vi "XML_value_to_variant.vi"(0 "XML-param":string) -> (1 "ParsingErrors":string, 2 "Value":variant, 3 "Type":T1(ring))   [LabVIEW 2010]
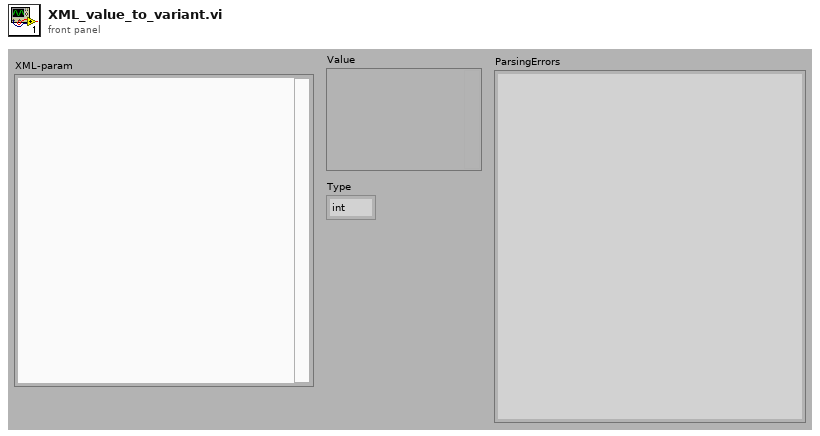
[diagram p1: front panel]
types:
  T1 = enum16{"int", "boolean", "string", "double", "dateTime", "base64", "struct", "array"}
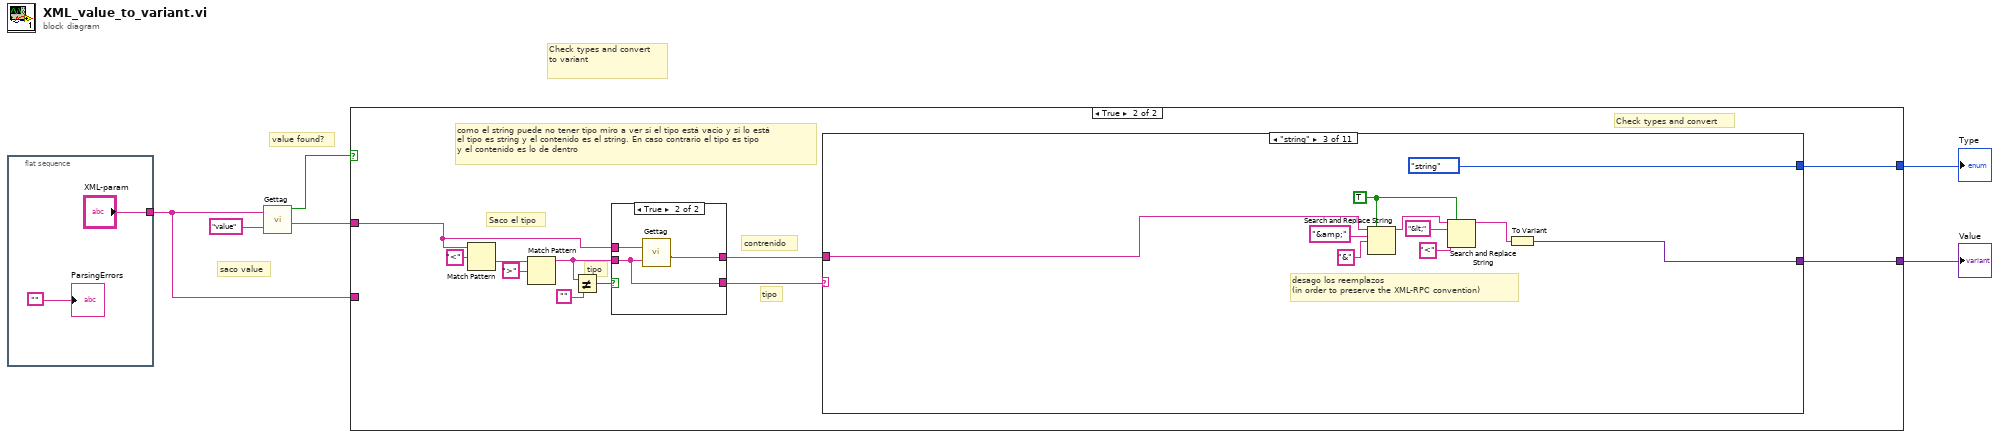
[diagram p0: block diagram]
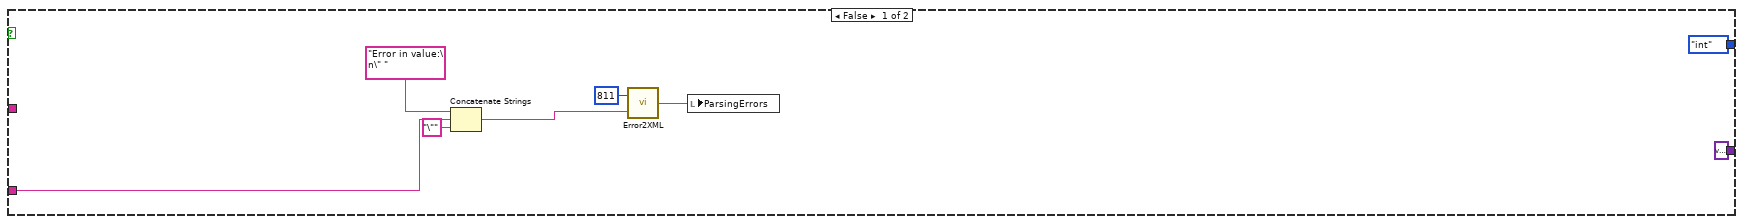
[diagram p2: hidden frame]
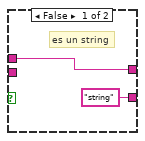
[diagram p3: hidden frame]
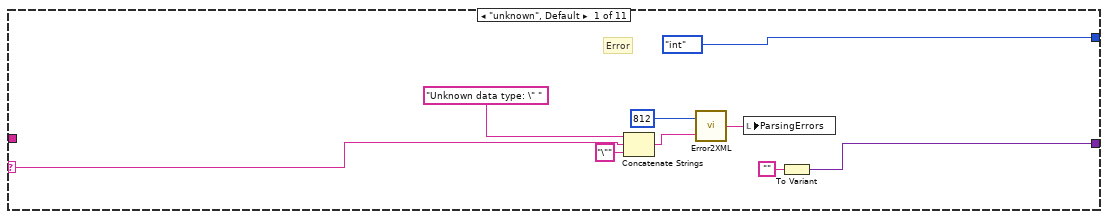
[diagram p4: hidden frame]
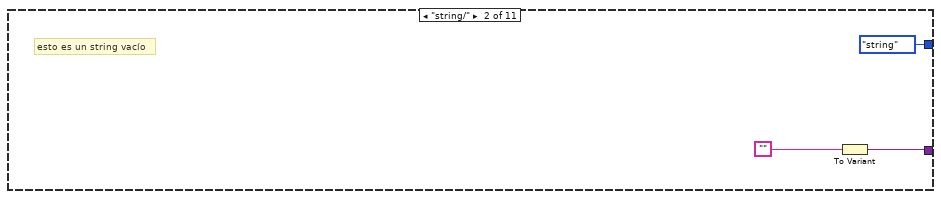
[diagram p5: hidden frame]
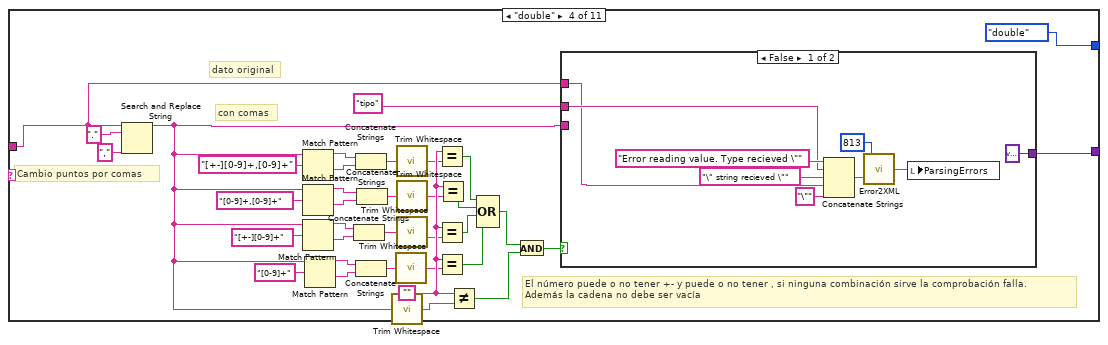
[diagram p6: hidden frame]
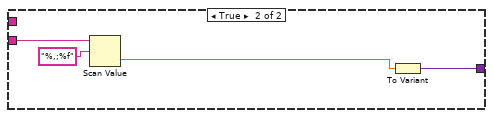
[diagram p7: hidden frame]
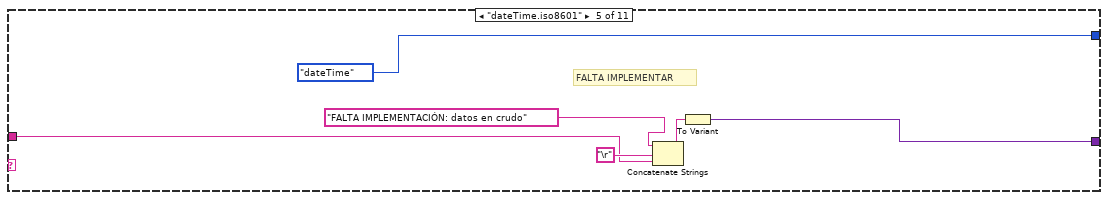
[diagram p8: hidden frame]
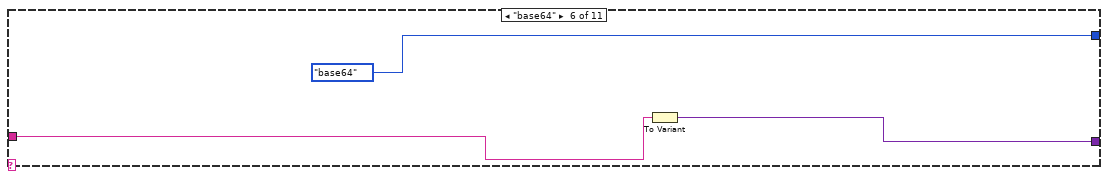
[diagram p9: hidden frame]
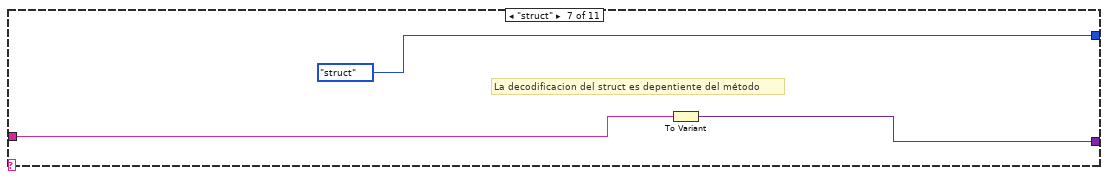
[diagram p10: hidden frame]
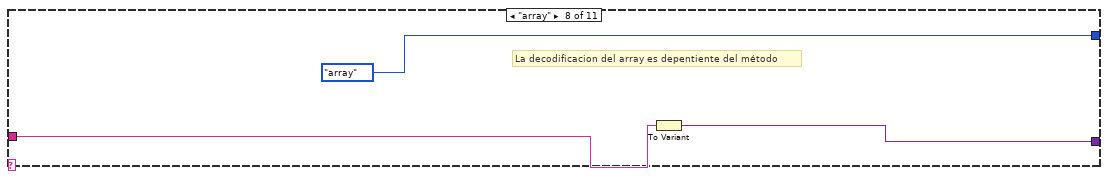
[diagram p11: hidden frame]
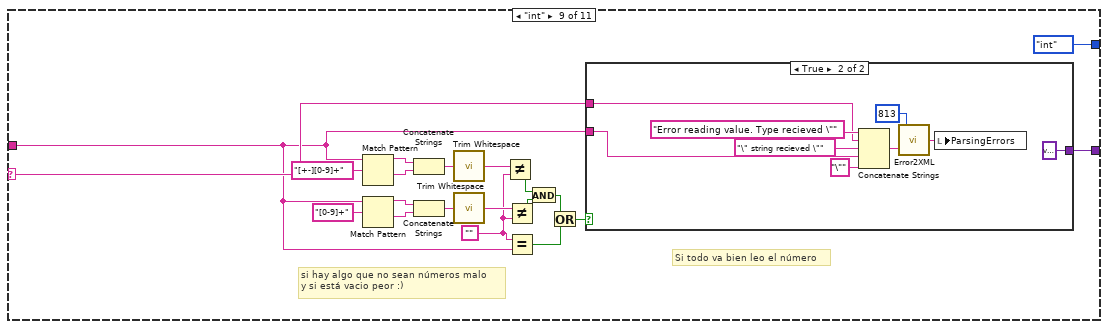
[diagram p12: hidden frame]
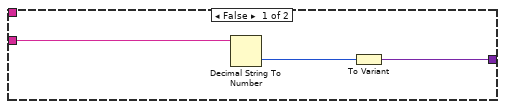
[diagram p13: hidden frame]
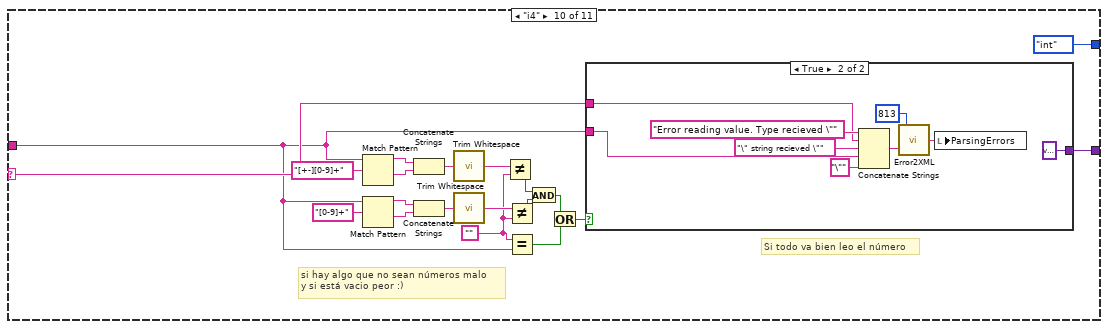
[diagram p14: hidden frame]
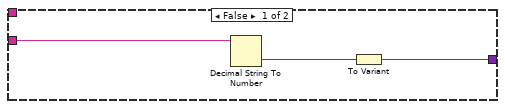
[diagram p15: hidden frame]
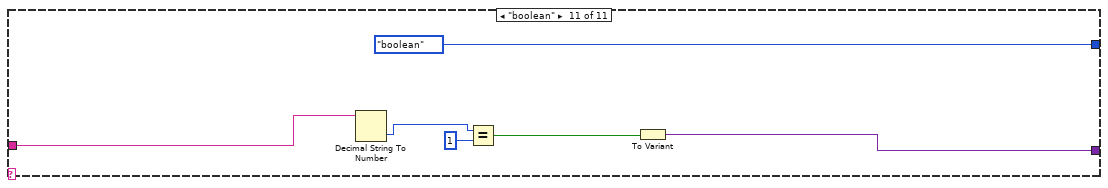
[diagram p16: hidden frame]
diagram:
  # "value found?"
  # "saco value"
  # "Check types and convert\nto variant"
  n1 = flat-sequence {
    tunnel: ["XML-param"] -> w3
    frame #0 {
      "ParsingErrors" <- ""
    }
  }
  n2 = call "Gettag.vi"("TagName"="value" ("regular expression"), "XML"=w3) -> ("InsideTag"=w1:string, "Found?"=w2:bool)  [unwired: 2 out]
  n3 = case shown="True" w2 {
    tunnel: [T1."int" w27] -> w6
    tunnel: [variant ("Variant") w26] -> w5
    tunnel: w3 -> [w9 _]
    tunnel: w1 -> [_ w22]
    frame False {
      n4 = Concatenate Strings("Error in value:\n\" ", w9, "\"" ("string")) -> (w12:string)
      n5 = call "Error2XML.vi"("FailDescriptor"=w12, "FailID"=811) -> ("ErrorXML"=w13:string)
      n6 = local write "ParsingErrors"(w13) -> ()
    }
    frame True {
      # "tipo"
      # "como el string puede no tener tipo miro a ver si el tipo está vacío y si lo está\nel tipo es string y el contenido es el string. En caso contrario el tipo es tipo \ny el contenido es lo de dentro"
      # "tipo"
      # "contrenido"
      # "Saco el tipo"
      # "Check types and convert"
      n7 = Match Pattern(string=w22, regular expression="<") -> (after substring=w24:string)  [unwired: 1 in, 3 out]
      n8 = Match Pattern(string=w24, regular expression=">") -> (before substring=w21:string)  [unwired: 1 in, 3 out]
      n9 = Not Equal?(x=w21, y="") -> (x != y?=w19:bool)
      n10 = case shown="True" w19 {
        tunnel: [w28 w32] -> w17
        tunnel: w22 -> [w28 w31]
        tunnel: w21 -> [_ w30]
        tunnel: ["string" ("InsideTag") w30] -> w18
        frame False {
          # "es un string"
        }
        frame True {
          n11 = call "Gettag.vi"("TagName"=w30, "XML"=w31) -> ("InsideTag"=w32:string)  [unwired: 3 out]
        }
      }
      n12 = case shown="\"string\"" w18 {
        selector: w18 -> [w33 _ _ _ _ _ _ _ w133 w165 _]
        tunnel: [T1."int" T1."string" T1."string" T1."double" T1."dateTime" T1."base64" T1."struct" T1."array" T1."int" T1."int" T1."boolean"] -> w27
        tunnel: w17 -> [_ _ w47 w56 w104 w110 w113 w116 w120 w152 w184]
        tunnel: [w35 w43 w49 w55 w105 w111 w114 w117 w125 w157 w185] -> w26
        frame "unknown", Default {
          # "Error"
          n13 = Concatenate Strings("Unknown data type: \" " ("FailDescriptor"), w33, "\"" ("string")) -> (w37:string)
          n14 = call "Error2XML.vi"("FailDescriptor"=w37, "FailID"=812) -> ("ErrorXML"=w36:string)
          n15 = local write "ParsingErrors"(w36) -> ()
          n16 = To Variant(anything="") -> (Variant=w35:variant)
        }
        frame "string/" {
          # "esto es un string vacío"
          n17 = To Variant(anything="") -> (Variant=w43:variant)
        }
        frame "string" {
          w46 = TRUE
          # "desago los reemplazos\n(in order to preserve the XML-RPC convention)"
          n18 = Search and Replace String(replace all?=w46, input string=w47, search string="&amp;" ("replace string (\"\")"), replace string="&" ("search string")) -> (result string=w45:string)  [unwired: 4 in, 3 out]
          n19 = Search and Replace String(replace all?=w46, input string=w45, search string="&lt;", replace string="<" ("replace string (\"\")")) -> (result string=w48:string)  [unwired: 4 in, 3 out]
          n20 = To Variant(anything=w48) -> (Variant=w49:variant)
        }
        frame "double" {
          w85 = ""
          # "con comas"
          # "El número puede o no tener +- y puede o no tener , si ninguna combinación sirve la comprobación falla.\nAdemás la cadena no debe ser vacía"
          # "dato original"
          # "Cambio puntos por comas"
          n21 = Search and Replace String(input string=w56, search string=".", replace string="," ("replace string (\"\")")) -> (result string=w57:string)  [unwired: 5 in, 3 out]
          n22 = Match Pattern(string=w57, regular expression="[+-][0-9]+,[0-9]+") -> (before substring=w62:string, after substring=w61:string)  [unwired: 1 in, 2 out]
          n23 = Match Pattern(string=w57, regular expression="[0-9]+,[0-9]+") -> (before substring=w66:string, after substring=w65:string)  [unwired: 1 in, 2 out]
          n24 = Match Pattern(string=w57, regular expression="[+-][0-9]+") -> (before substring=w74:string, after substring=w73:string)  [unwired: 1 in, 2 out]
          n25 = Match Pattern(string=w57, regular expression="[0-9]+") -> (before substring=w70:string, after substring=w69:string)  [unwired: 1 in, 2 out]
          n26 = Concatenate Strings(w74, w73) -> (w72:string)
          n27 = Concatenate Strings(w62, w61) -> (w60:string)
          n28 = Concatenate Strings(w70, w69) -> (w68:string)
          n29 = Concatenate Strings(w66, w65) -> (w64:string)
          n30 = call <vilib>:"Trim Whitespace.vi"("string"=w57) -> ("trimmed string"=w86:string)  [unwired: 1 in]
          n31 = call <vilib>:"Trim Whitespace.vi"("string"=w68) -> ("trimmed string"=w76:string)  [unwired: 1 in]
          n32 = call <vilib>:"Trim Whitespace.vi"("string"=w60) -> ("trimmed string"=w79:string)  [unwired: 1 in]
          n33 = call <vilib>:"Trim Whitespace.vi"("string"=w64) -> ("trimmed string"=w78:string)  [unwired: 1 in]
          n34 = call <vilib>:"Trim Whitespace.vi"("string"=w72) -> ("trimmed string"=w77:string)  [unwired: 1 in]
          n35 = Equal?(x=w85, y=w79) -> (x = y?=w80:bool)
          n36 = Equal?(x=w85, y=w77) -> (x = y?=w82:bool)
          n37 = Equal?(x=w85, y=w76) -> (x = y?=w83:bool)
          n38 = Equal?(x=w85, y=w78) -> (x = y?=w81:bool)
          n39 = Not Equal?(x=w85, y=w86) -> (x != y?=w87:bool)
          n40 = Compound Arithmetic op=OR(w80, w81, w82, w83) -> (w84:bool)
          n41 = And(x=w84, y=w87) -> (x .and. y?=w59:bool)
          n42 = case shown="False" w59 {
            tunnel: "tipo" ("format string") -> [w94 _]
            tunnel: w57 -> [_ w102]
            tunnel: w56 -> [w93 _]
            tunnel: [variant ("Variant") w101] -> w55
            frame False {
              n43 = Concatenate Strings("Error reading value. Type recieved \"" ("string"), w94, "\" string recieved \"" ("string"), w93, "\"" ("string")) -> (w99:string)
              n44 = call "Error2XML.vi"("FailDescriptor"=w99, "FailID"=813) -> ("ErrorXML"=w92:string)
              n45 = local write "ParsingErrors"(w92) -> ()
            }
            frame True {
              n46 = Scan Value(string=w102, format string="%,;%f") -> (value=w100:dbl)  [unwired: 1 in, 1 out]
              n47 = To Variant(anything=w100) -> (Variant=w101:variant)
            }
          }
        }
        frame "dateTime.iso8601" {
          # "FALTA IMPLEMENTAR"
          n48 = Concatenate Strings("FALTA IMPLEMENTACIÓN: datos en crudo", "\r", w104) -> (w106:string)
          n49 = To Variant(anything=w106) -> (Variant=w105:variant)
        }
        frame "base64" {
          n50 = To Variant(anything=w110) -> (Variant=w111:variant)
        }
        frame "struct" {
          # "La decodificacion del struct es depentiente del método"
          n51 = To Variant(anything=w113) -> (Variant=w114:variant)
        }
        frame "array" {
          # "La decodificacion del array es depentiente del método"
          n52 = To Variant(anything=w116) -> (Variant=w117:variant)
        }
        frame "int" {
          w121 = ""
          # "Si todo va bien leo el número"
          # "si hay algo que no sean números malo\ny si está vacio peor :)"
          n53 = Match Pattern(string=w120, regular expression="[+-][0-9]+") -> (before substring=w136:string, after substring=w135:string)  [unwired: 1 in, 2 out]
          n54 = Match Pattern(string=w120, regular expression="[0-9]+") -> (before substring=w131:string, after substring=w130:string)  [unwired: 1 in, 2 out]
          n55 = Concatenate Strings(w136, w135) -> (w134:string)
          n56 = Concatenate Strings(w131, w130) -> (w129:string)
          n57 = call <vilib>:"Trim Whitespace.vi"("string"=w134) -> ("trimmed string"=w128:string)  [unwired: 1 in]
          n58 = call <vilib>:"Trim Whitespace.vi"("string"=w129) -> ("trimmed string"=w127:string)  [unwired: 1 in]
          n59 = Not Equal?(x=w128, y=w121) -> (x != y?=w126:bool)
          n60 = Not Equal?(x=w127, y=w121) -> (x != y?=w124:bool)
          n61 = Equal?(x=w121, y=w120) -> (x = y?=w122:bool)
          n62 = And(x=w126, y=w124) -> (x .and. y?=w123:bool)
          n63 = Or(x=w123, y=w122) -> (x .or. y?=w119:bool)
          n64 = case shown="True" w119 {
            tunnel: w133 -> [_ w145]
            tunnel: w120 -> [w141 w144]
            tunnel: [w139 variant ("Variant")] -> w125
            frame False {
              n65 = Decimal String To Number(string=w141) -> (number=w140:i32)  [unwired: 2 in, 1 out]
              n66 = To Variant(anything=w140) -> (Variant=w139:variant)
            }
            frame True {
              n67 = Concatenate Strings("Error reading value. Type recieved \"" ("string"), w145, "\" string recieved \"" ("string"), w144, "\"" ("string")) -> (w149:string)
              n68 = call "Error2XML.vi"("FailDescriptor"=w149, "FailID"=813) -> ("ErrorXML"=w150:string)
              n69 = local write "ParsingErrors"(w150) -> ()
            }
          }
        }
        frame "i4" {
          w153 = ""
          # "Si todo va bien leo el número"
          # "si hay algo que no sean números malo\ny si está vacio peor :)"
          n70 = Match Pattern(string=w152, regular expression="[+-][0-9]+") -> (before substring=w168:string, after substring=w167:string)  [unwired: 1 in, 2 out]
          n71 = Match Pattern(string=w152, regular expression="[0-9]+") -> (before substring=w163:string, after substring=w162:string)  [unwired: 1 in, 2 out]
          n72 = Concatenate Strings(w168, w167) -> (w166:string)
          n73 = Concatenate Strings(w163, w162) -> (w161:string)
          n74 = call <vilib>:"Trim Whitespace.vi"("string"=w166) -> ("trimmed string"=w160:string)  [unwired: 1 in]
          n75 = call <vilib>:"Trim Whitespace.vi"("string"=w161) -> ("trimmed string"=w159:string)  [unwired: 1 in]
          n76 = Not Equal?(x=w160, y=w153) -> (x != y?=w158:bool)
          n77 = Not Equal?(x=w159, y=w153) -> (x != y?=w156:bool)
          n78 = Equal?(x=w153, y=w152) -> (x = y?=w154:bool)
          n79 = And(x=w158, y=w156) -> (x .and. y?=w155:bool)
          n80 = Or(x=w155, y=w154) -> (x .or. y?=w151:bool)
          n81 = case shown="True" w151 {
            tunnel: w165 -> [_ w177]
            tunnel: w152 -> [w173 w176]
            tunnel: [w171 variant ("Variant")] -> w157
            frame False {
              n82 = Decimal String To Number(string=w173) -> (number=w172:i32)  [unwired: 2 in, 1 out]
              n83 = To Variant(anything=w172) -> (Variant=w171:variant)
            }
            frame True {
              n84 = Concatenate Strings("Error reading value. Type recieved \"" ("string"), w177, "\" string recieved \"" ("string"), w176, "\"" ("string")) -> (w181:string)
              n85 = call "Error2XML.vi"("FailDescriptor"=w181, "FailID"=813) -> ("ErrorXML"=w182:string)
              n86 = local write "ParsingErrors"(w182) -> ()
            }
          }
        }
        frame "boolean" {
          n87 = Decimal String To Number(string=w184) -> (number=w183:i32)  [unwired: 2 in, 1 out]
          n88 = Equal?(x=w183, y=1) -> (x = y?=w186:bool)
          n89 = To Variant(anything=w186) -> (Variant=w185:variant)
        }
      }
    }
  }
  "Type" <- w6
  "Value" <- w5
